vi "Initialise Texture From File.vi"(6 "Scale":sgl=1.0, 7 "Renderer":u32, 8 "error in (no error)":errorcluster, 10 "Name":string, 11 "File":path) -> (0 "error out":errorcluster, 3 "Name In Cache":string)   [LabVIEW 2021, in "Resource Manager.lvclass"]
uses:
  Resource Manager.lvclass
  Resource Manager.lvclass/Resource Manager.ctl
  Texture/Texture.lvclass
  Globals.vi
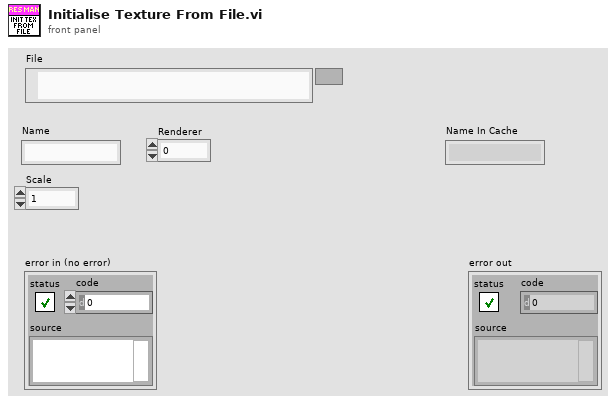
[diagram p1: front panel]
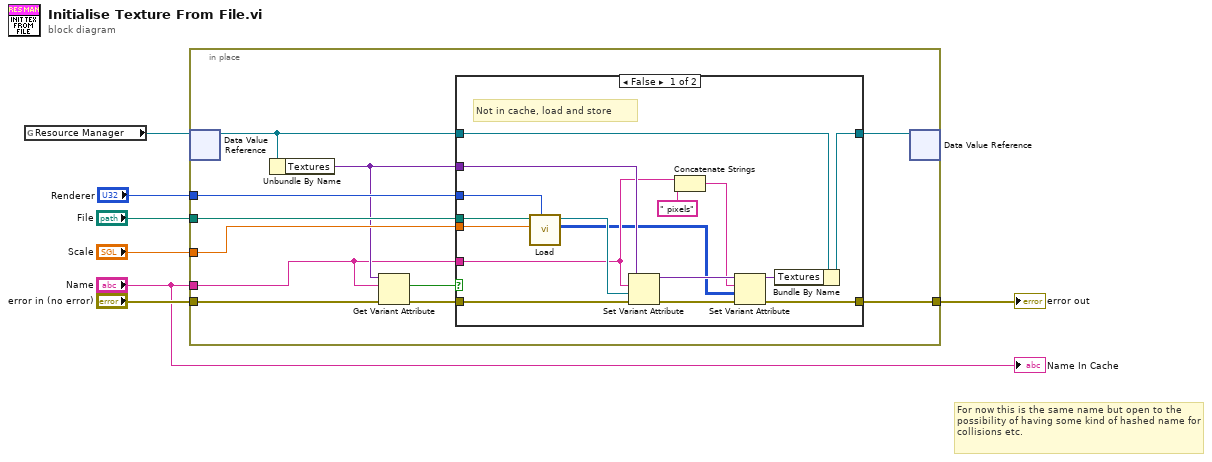
[diagram p0: block diagram]
diagram:
  # "For now this is the same name but open to the possibility of having some kind of hashed name for collisions etc."
  n1 = global read "Globals.vi" "Resource Manager"() -> (w2:refnum<data-value>)
  n2 = in-place {
    in-place-border: "File" -> [w15]
    in-place-border: "Scale" -> [w14]
    in-place-border: "error in (no error)" -> [w11]
    in-place-border: [w18] -> w4
    in-place-border: "Name" -> [w9]
    in-place-border: "Renderer" -> [w13]
    n3 = in-place-dvr #1(w2) -> (w17:refnum<class "Resource Manager.lvclass">)  [unwired: 1 out]
    n4 = Unbundle By Name(w17) -> ("Textures"=w10:variant)
    n5 = Get Variant Attribute(Variant=w10, name=w9, error in=w11) -> (found=w8:bool, error out=w12:errorcluster)  [unwired: 1 in, 2 out]
    n6 = case shown="False" w8 {
      tunnel: [w25 w35] -> w18
      tunnel: w17 -> [w33 w36]
      tunnel: [w32 w36] -> w16
      tunnel: w15 -> [w31 _]
      tunnel: w14 -> [w30 _]
      tunnel: w13 -> [w29 _]
      tunnel: w12 -> [w28 w35]
      tunnel: w10 -> [w27 _]
      tunnel: w9 -> [w22 _]
      frame False {
        # "Not in cache, load and store"
        n7 = call "Load.vi"("Renderer"=w29, "Scale"=w30, "Path"=w31) -> ("Pixels"=w19:u32[][], "Texture out"=w34:refnum<class "Texture.lvclass">)  [unwired: 6 in, 1 out]
        n8 = Set Variant Attribute(Variant=w27, name=w22, value=w34, error in=w28) -> (Variant out=w24:variant, error out=w26:errorcluster)  [unwired: 1 out]
        n9 = Concatenate Strings(w22, " pixels" ("string")) -> (w20:string)
        n10 = Set Variant Attribute(Variant=w24, name=w20, value=w19, error in=w26) -> (Variant out=w23:variant, error out=w25:errorcluster)  [unwired: 1 out]
        n11 = Bundle By Name(cluster=w33, "Textures"=w23) -> (w32:refnum<class "Resource Manager.lvclass">)
      }
      frame True {
        # "Already in cache. No need to re-add"
      }
    }
    n12 = in-place-dvr #1(w16) -> ()  [unwired: 2 out]
  }
  "error out" <- w4
  "Name In Cache" <- "Name"
